vi "Control Loop vthreshold.vi"() -> ()   [LabVIEW 2018]
uses:
  6dd9ee85-ba6e-44a8-aef2-e5238686a65b.vi
  5806a1ee-71b2-4ad4-b6eb-d772d2e731e4.vi
  <vilib>/Plasmionique/MB Master/MB_Master_TCP/MB_Master_TCP.lvclass
  C:/Program Files (x86)/National Instruments/LabVIEW 2018/vi.lib/Plasmionique/MB Master/MB_Master/MB_Master.lvclass
  <vilib>/Plasmionique/MB Master/MB Master.lvlib
panel:
  in  "Curtailment %":u16
  in  "IP Address":string="localhost"
  in  "stop":bool
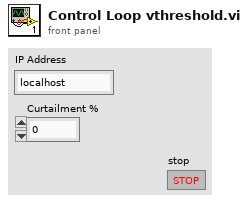
[diagram p1: front panel]
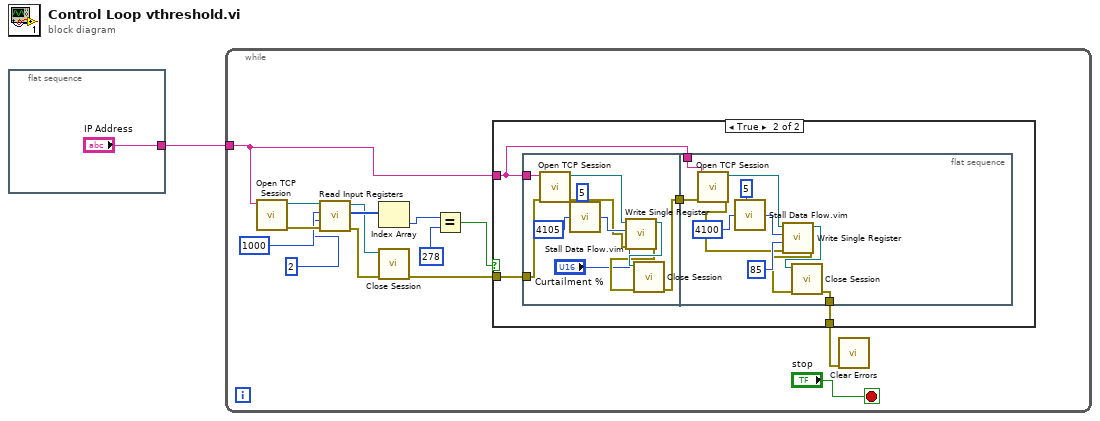
[diagram p0: block diagram]
diagram:
  n1 = flat-sequence {
    tunnel: ["IP Address"] -> w1
    frame #0 {
    }
  }
  n2 = while {
    tunnel: w1 -> [w13]
    stop <- "stop" stop-if-true
    n3 = call <vilib>:"Open TCP Session.vi"("IP Address"=w13) -> ("error out"=w9:errorcluster, "MB_TCP session"=w10:refnum<class "MB_Master_TCP.lvclass">)  [unwired: 9 in]
    n4 = call <vilib>:"Read Input Registers.vi"("error in (no error)"=w9, "quantity"=u16 2, "starting address"=u16 1000 ("quantity"), "MB session in"=w10) -> ("error out"=w8:errorcluster, "Registers"=w7:u16[], "MB session out"=w6:refnum<class "MB_Master_TCP.lvclass">)  [unwired: 5 in]
    n5 = Index Array(array=w7) -> (element=w3:u16)  [unwired: 1 in]
    n6 = call-dynamic "Close Session.vi"("error in (no error)"=w8, "MB TCP session"=w6) -> ("error out"=w12:errorcluster)  [unwired: 9 in]
    n7 = Equal?(x=w3, y=u16 278) -> (x = y?=w14:bool)
    n8 = case shown="True" w14 {
      tunnel: w13 -> [_ w20]
      tunnel: w12 -> [_ w19]
      tunnel: [_ w17] -> w11
      frame False {
      }
      frame True {
        n9 = flat-sequence {
          tunnel: w20 -> [w31]
          tunnel: w19 -> [w25]
          tunnel: [w22] -> w18
          tunnel: w20 -> [w42]
          tunnel: w18 -> [w35]
          tunnel: [w32] -> w17
          frame #0 {
            n10 = call <vilib>:"Open TCP Session.vi"("error in (no error)"=w25, "IP Address"=w31) -> ("error out"=w24:errorcluster, "MB_TCP session"=w30:refnum<class "MB_Master_TCP.lvclass">)  [unwired: 8 in]
            n11 = call "Stall Data Flow.vim"("value in"=u16 4105 ("address"), "milliseconds to wait"=u32 5) -> ("value out"=w26:u16)  [unwired: 1 out]
            n12 = call <vilib>:"Write Single Register.vi"("error in (no error)"=w24, "value"="Curtailment %", "address"=w26, "MB session in"=w30) -> ("error out"=w23:errorcluster, "MB session out"=w29:refnum<class "MB_Master_TCP.lvclass">)  [unwired: 6 in]
            n13 = call-dynamic "Close Session.vi"("error in (no error)"=w23, "MB TCP session"=w29) -> ("error out"=w22:errorcluster)  [unwired: 9 in]
          }
          frame #1 {
            n14 = call <vilib>:"Open TCP Session.vi"("error in (no error)"=w35, "IP Address"=w42) -> ("error out"=w34:errorcluster, "MB_TCP session"=w41:refnum<class "MB_Master_TCP.lvclass">)  [unwired: 8 in]
            n15 = call "Stall Data Flow.vim"("value in"=u16 4100 ("address"), "milliseconds to wait"=u32 5) -> ("value out"=w37:u16)  [unwired: 1 out]
            n16 = call <vilib>:"Write Single Register.vi"("error in (no error)"=w34, "value"=u16 85, "address"=w37, "MB session in"=w41) -> ("error out"=w33:errorcluster, "MB session out"=w40:refnum<class "MB_Master_TCP.lvclass">)  [unwired: 6 in]
            n17 = call-dynamic "Close Session.vi"("error in (no error)"=w33, "MB TCP session"=w40) -> ("error out"=w32:errorcluster)  [unwired: 9 in]
          }
        }
      }
    }
    n18 = call <vilib>:"Clear Errors.vi"("error in (no error)"=w11) -> ()  [unwired: 5 in, 2 out]
  }
